vi "Bind Terminal Value.vi"(4 "Ignore Past Updates? (F)":bool, 6 "Value Changes Only? (T)":bool=TRUE, 8 "error in (no error)":errorcluster, 9 "Datum Name (\"\"=Use Control Label)":string, 10 "Ctl Refnum":refnum<vi>, 11 "IObserver in":refnum<class "IObserver.lvclass">) -> (0 "error out":errorcluster, 3 "IObserver out":refnum<class "IObserver.lvclass">)   [LabVIEW 2015, in "IObserver.lvlib" / "IObserver.lvclass"]
doc: "<License>\nCopyright © 2017 Composed Systems, LLC | All rights reserved\nwww.composed.io\n\nAuthor: Ethan Stern <ethan.stern@composed.io>\n\nThis software is provided \"AS IS\" WITHOUT WARRANTIES, either express or implied, AND IS FOR EDUCATIONAL PURPOSES ONLY.\n</License>"
uses:
  IObserver.lvclass
  <vilib>/ActorFramework/Actor/Actor.lvclass/Actor.ctl
  <vilib>/ActorFramework/Message Enqueuer/Message Enqueuer.lvclass/Message Enqueuer.ctl
  SubscriptionPolicy/BasicSubscription/BasicSubscription.lvclass/BasicSubscription.ctl
  SubscriptionPolicy/ValueChangeSubscription/ValueChangeSubscription.lvclass/ValueChangeSubscription.ctl
  IObserver Messages/Subscribe Msg/Subscribe Msg.lvclass/Subscribe Msg.ctl
  <vilib>/ActorFramework/Message Enqueuer/Init from Existing Queue.vi
  <vilib>/ActorFramework/Message Enqueuer/Enqueue.vi
  <vilib>/ActorFramework/Message Priority Queue/Priority Enqueue.vi
  <vilib>/ActorFramework/Message Enqueuer/Message Enqueuer.lvclass
  SubscriptionPolicy/BasicSubscription/BasicSubscription.lvclass
  SubscriptionPolicy/ValueChangeSubscription/ValueChangeSubscription.lvclass
  IObserver Messages/Subscribe Msg/Subscribe Msg.lvclass
  IMediator/SubscriptionRequest/SubscriptionRequest.lvclass
  <vilib>/ActorFramework/Actor/Actor.lvclass
  Transport/TerminalBinding/TerminalBinding.lvclass
  IMediator/ISubscriptionPolicy/ISubscriptionPolicy.lvclass
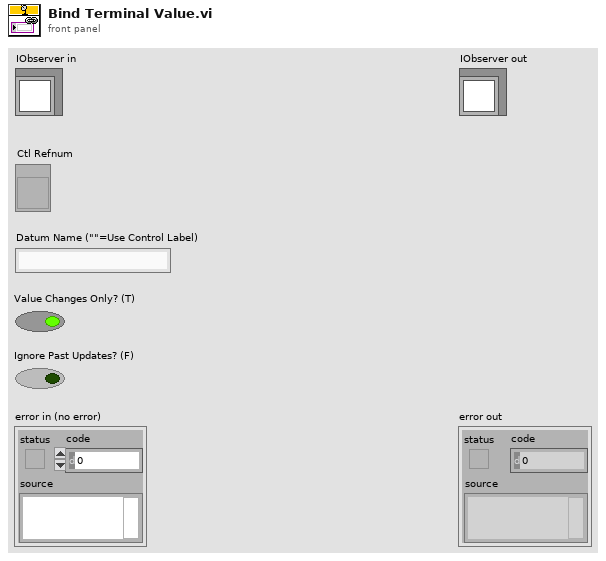
[diagram p1: front panel]
types:
  T1 = typedef "IMediator.lvlib/ISubscriptionPolicy.lvclass/ISubscriptionPolicy Reference.ctl" = refnum<data-value>
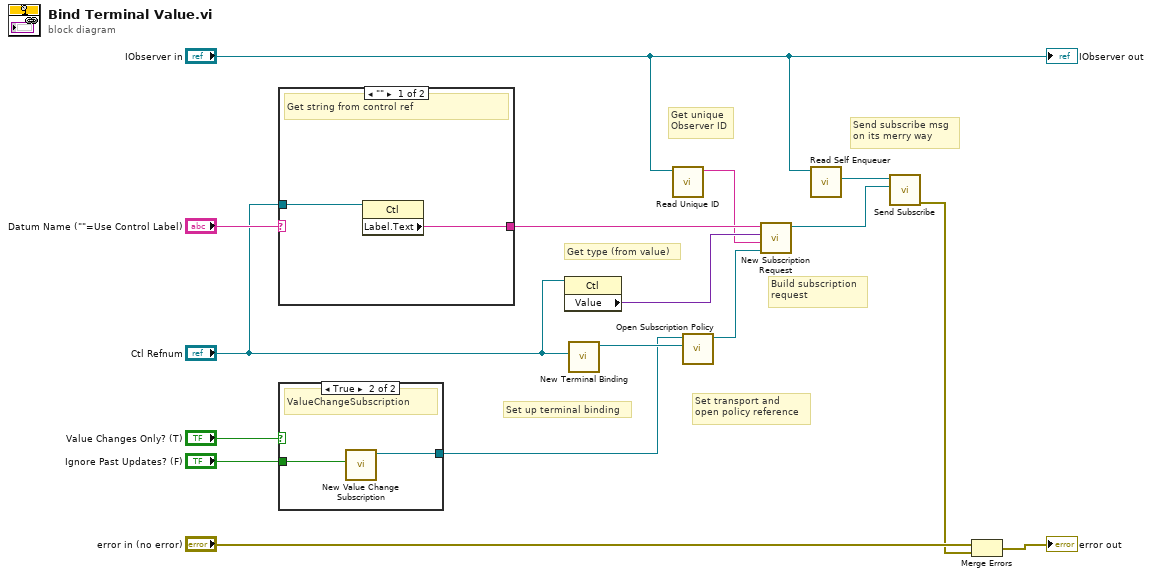
[diagram p0: block diagram]
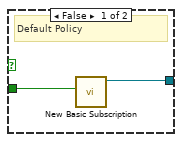
[diagram p2: hidden frame]
diagram:
  # "Set transport and\nopen policy reference"
  # "Send subscribe msg\non its merry way"
  # "Build subscription\nrequest"
  # "Get unique\nObserver ID"
  # "Get type (from value)"
  # "Set up terminal binding"
  n1 = case shown="\"\"" "Datum Name (\"\"=Use Control Label)" {
    selector: "Datum Name (\"\"=Use Control Label)" -> [_ w19]
    tunnel: [w17 w19] -> w8
    tunnel: "Ctl Refnum" -> [w18 _]
    frame "" {
      # "Get string from control ref"
      n2 = property class="Ctl"(reference=w18) -> ("Label.Text"=w17:string)  [unwired: 1 in, 2 out]
    }
    frame Default {
      # "Use string wired to input terminal"
    }
  }
  n3 = case shown="True" "Value Changes Only? (T)" {
    tunnel: "Ignore Past Updates? (F)" -> [w20 w23]
    tunnel: [w21 w22] -> w2
    frame False {
      # "Default Policy"
      n4 = call "New Basic Subscription.vi"("Ignore Past Updates? (F)"=w20) -> ("BasicSubscription Out"=w21:refnum<class "BasicSubscription.lvclass">)  [unwired: 10 in]
    }
    frame True {
      # "ValueChangeSubscription"
      n5 = call "New Value Change Subscription.vi"("Ignore Past Updates? (F)"=w23) -> ("ValueChangeSubscription Out"=w22:refnum<class "ValueChangeSubscription.lvclass">)  [unwired: 10 in]
    }
  }
  n6 = property class="Ctl"(reference="Ctl Refnum") -> ("Value"=w15:variant)  [unwired: 1 in, 2 out]
  n7 = call "New Terminal Binding.vi"("Ctl Refnum"="Ctl Refnum") -> ("TerminalBinding"=w5:refnum<class "TerminalBinding.lvclass">)  [unwired: 9 in, 1 out]
  n8 = call "Read Unique ID.vi"("IObserver In"="IObserver in") -> ("Unique ID"=w4:string)  [unwired: 10 in]
  n9 = call "Open Subscription Policy.vi"("Transport"=w5, "SubscriptionPolicy"=w2) -> ("Subscription Policy"=w6:T1)  [unwired: 8 in, 1 out]
  n10 = call "New Subscription Request.vi"("Subscription Policy"=w6, "Subscriber ID"=w4, "Type"=w15, "Datum Name"=w8) -> ("SubscriptionRequest"=w12:refnum<class "SubscriptionRequest.lvclass">)  [unwired: 7 in]
  n11 = call <vilib>:"Read Self Enqueuer.vi"("Actor"="IObserver in") -> ("Self Enqueuer"=w13:refnum<class "Message Enqueuer.lvclass">)  [unwired: 10 in]
  n12 = call "Send Subscribe.vi"("SubscriptionRequest"=w12, "Message Enqueuer"=w13) -> ("error out"=w10:errorcluster)  [unwired: 8 in, 1 out]
  n13 = Merge Errors("error in (no error)", w10) -> (→"error out":errorcluster)
  "IObserver out" <- "IObserver in"
